vi "CSM_ExampleBrowser.vi"() -> ()   [LabVIEW 2017, in "CSM_ExampleBrowser.lvlib"]
uses:
  CSM_ExampleBrowser.lvlib
  controls/BMark_UI Data.ctl
  <vilib>/addons/analyzer/_analyzerctrls.llb/VIAnCtl Analysis App Info.ctl
  controls/BMark_Bookmark Data.ctl
  controls/BMark_VI_Identifier.ctl
  <vilib>/event_ctls.llb/eventvkey.ctl
  <vilib>/Utility/miscctls.llb/LVPoint32TypeDef.ctl
  4b753ef9-0da6-4ee4-b2e8-a0e51625f9fb.vi
  <vilib>/Array/Sort 2D Array - Pop Stack.vi
  <vilib>/Array/Sort 2D Array - Push Stack.vi
  globals/BMark_User Visible Strings.vi
  <userlib>/_OpenG.lib/string/string.llb/Convert EOLs (String)__ogtk.vi
  _Shared/CSM Shared.lvlib
  Communicable State Machine.lvlib
  _Support/csm-tool-support.lvlib
panel:
  in  "BookmarkTree":string(tree)
  in  "Refresh":bool
  in  "Zoom Factor":dbl(slide)=0.1 min=0.1 max=1.0 step=0.001 scale=0.1..1.0
  out "Warning glyph":bool
  in  "ExampleTree":string(tree)
  in  "BookmarkList":i32(listbox)
  out "String":string
  out "Preview":picture
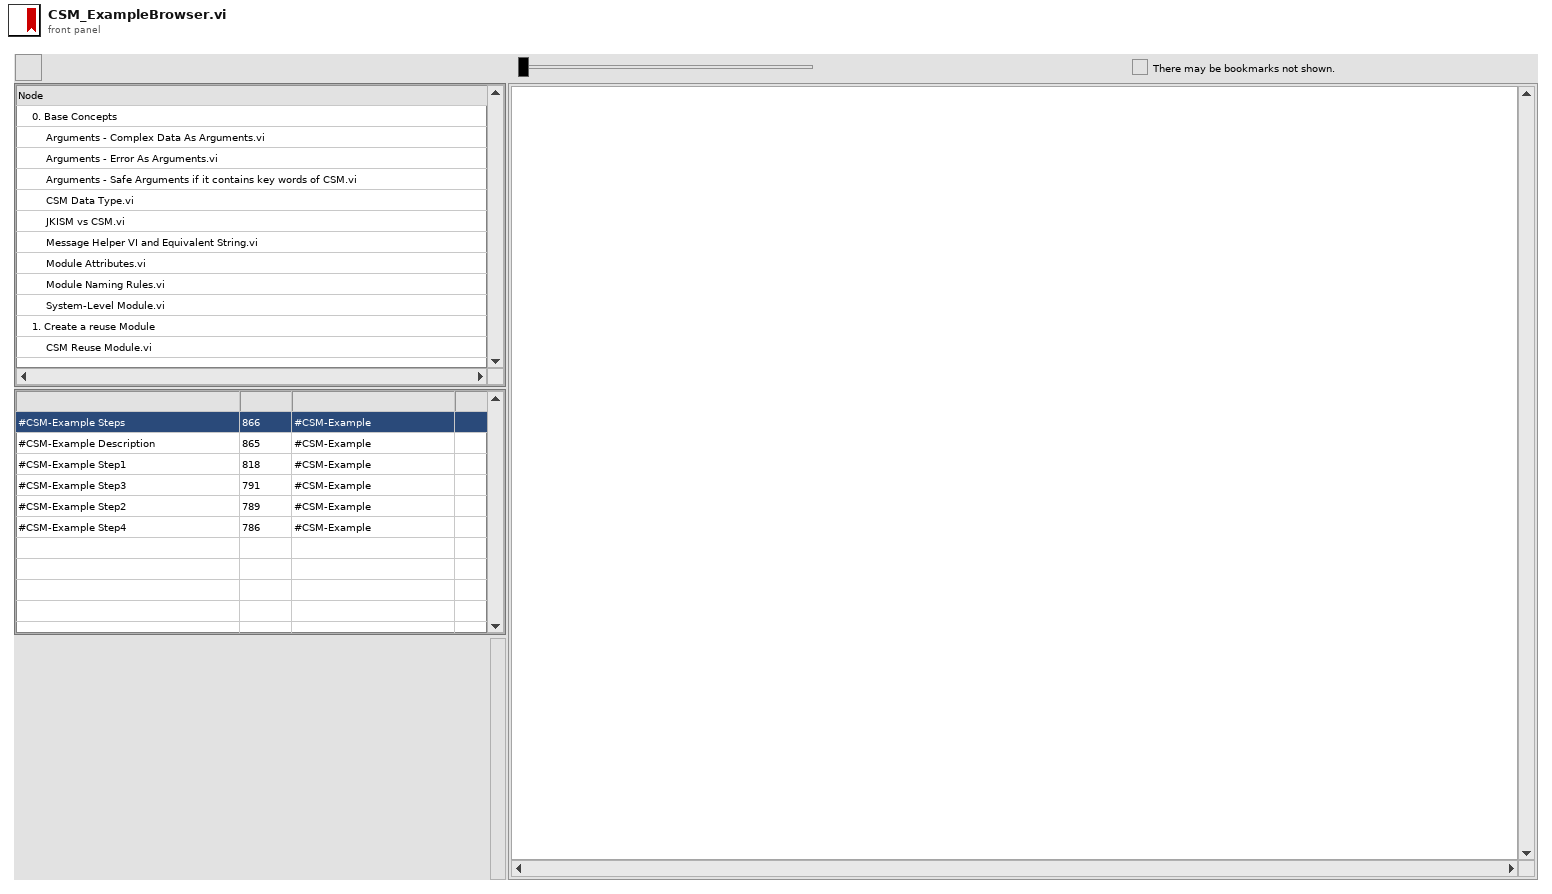
[diagram p1: front panel]
types:
  T1 = typedef "BMark_UI Data.ctl" = cluster{"Tree":refnum<vi>, "Warning glyph":refnum<vi>, "More information":refnum<vi>, "Front Panel":refnum<vi>, "GroupByVI":bool, "all projects":T2[], "bookmarks":T3[], "App Info":T2, "Preview image":refnum<vi>}
  T2 = typedef "VIAnCtl Analysis App Info.ctl" = cluster{"Project Name":string, "Target Name":string}
  T3 = typedef "BMark_Bookmark Data.ctl" = cluster{"bookmark tag":string, "full text":string, "bookmark ref":i32, "VI display name":string, "VI identifier":T4}
  T4 = typedef "BMark_VI_Identifier.ctl" = cluster{"Name":string, "Path":path, "App Info":T2}
  T5 = typedef "eventvkey.ctl" = enum16{"ASCII", "Enter", "Return", "Shift", "Ctrl", "Alt", "Cmd", "Opt", "Caps", "NumLock", "Clear", "Break", "Up", "Down", "Left", "Right", "Insert", "Delete", "Home", "End", "PageUp", "PageDown", "Escape", "Help", "Pause", "ScrollLock", "F1", "F2", "F3", "F4", "F5", "F6", "F7", "F8", "F9", "F10", "F11", "F12", "F13", "F14", "F15", "F16", "F17", "F18", "F19", "F20", "F21", "F22", "F23", "F24", "Play", "VolumeUp", "VolumeDown", "Mute", "Two Byte Char"}
  T6 = enum32{"Invalid", "Standard", "Closed", "Hidden", "Minimized", "Maximized"}
  T7 = enum32{"invalid app kind", "Development System", "Run Time System", "Student Edition", "Embedded LabVIEW", "Evaluation", "Custom"}
  T8 = enum8{"Enabled", "Disabled", "Disabled and Grayed Out"}
  T9 = typedef "LVPoint32TypeDef.ctl" = cluster{"Horizontal":i32, "Vertical":i32}
  T10 = typedef "LVPointTypeDef.ctl" = cluster{"Horizontal":i16, "Vertical":i16}
  T11 = cluster{"Core":cluster{"Current VI Reference":refnum<vi>, "Close Panel on Exit?":bool}, "root":path, "PreviewMouseDown":bool, "PreviewMouseDownCoords":T9, "PreviewMouseDownOrigin":T9}
  T12 = typedef "LVRectTypeDef.ctl" = cluster{"Left":i16, "Top":i16, "Right":i16, "Bottom":i16}
  T13 = cluster{"Current VI Reference":refnum<vi>, "Close Panel on Exit?":bool}
  T14 = typedef "LVBookmarkInfoTypeDef.ctl" = cluster{"Bookmark Reference":u32, "Bookmark Tag":string, "Label Text":string}[]
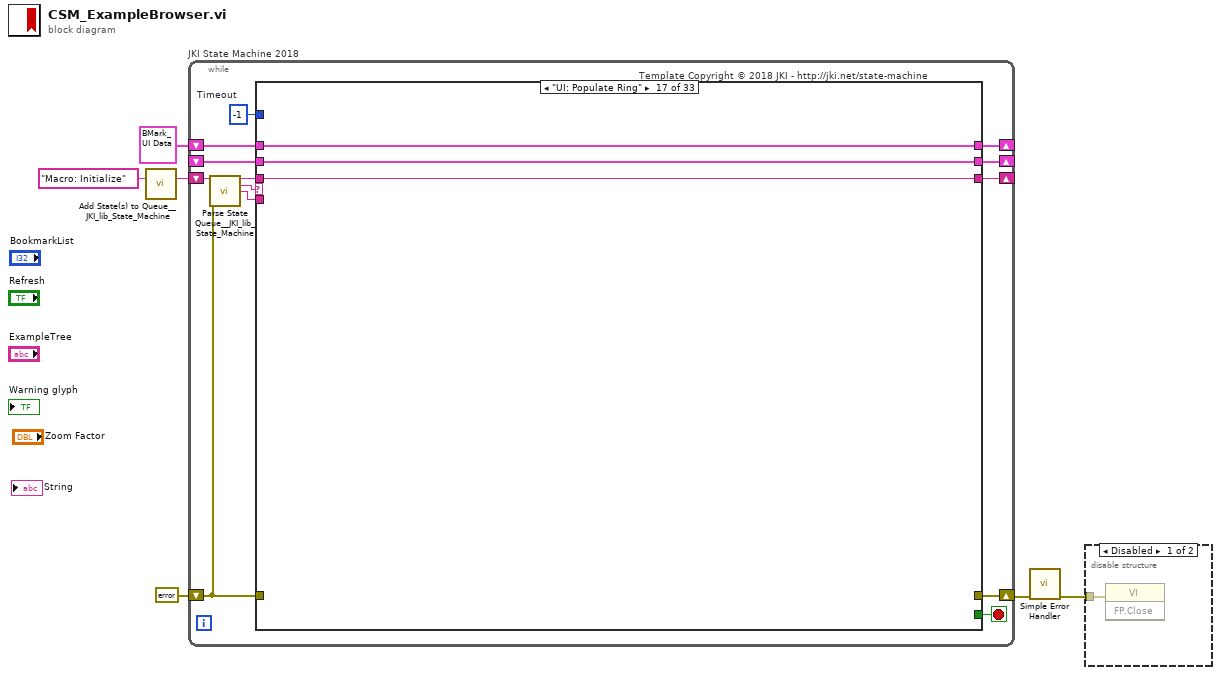
[diagram p0: block diagram]
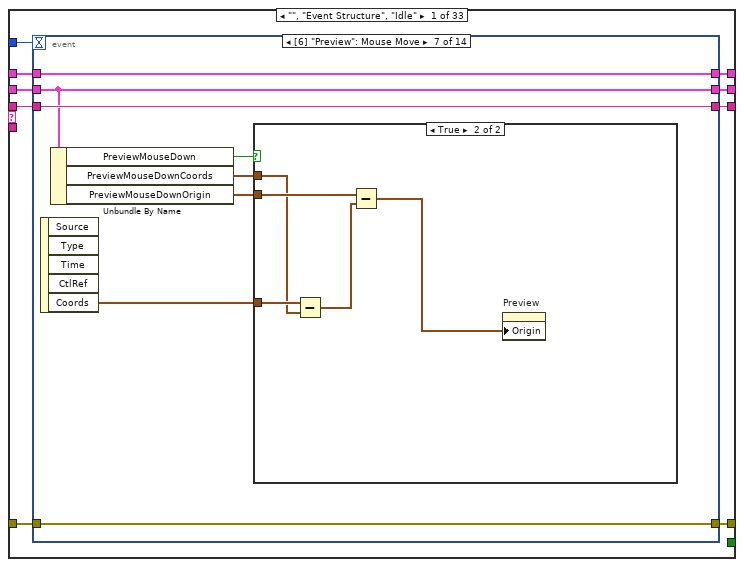
[diagram p2: hidden frame]
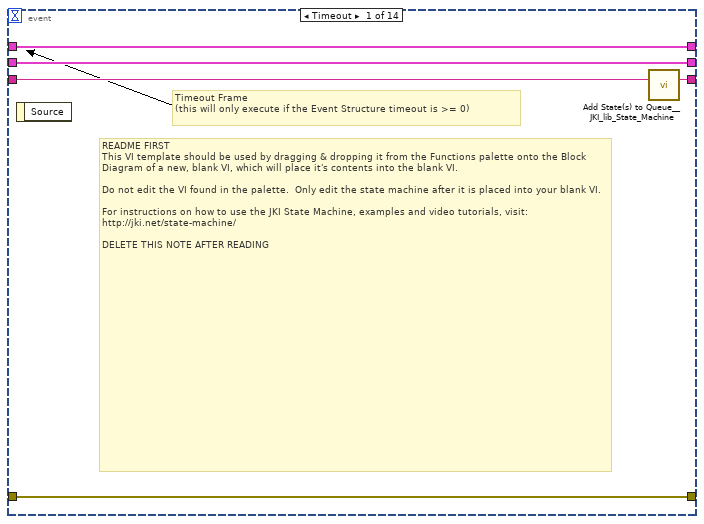
[diagram p3: hidden frame]
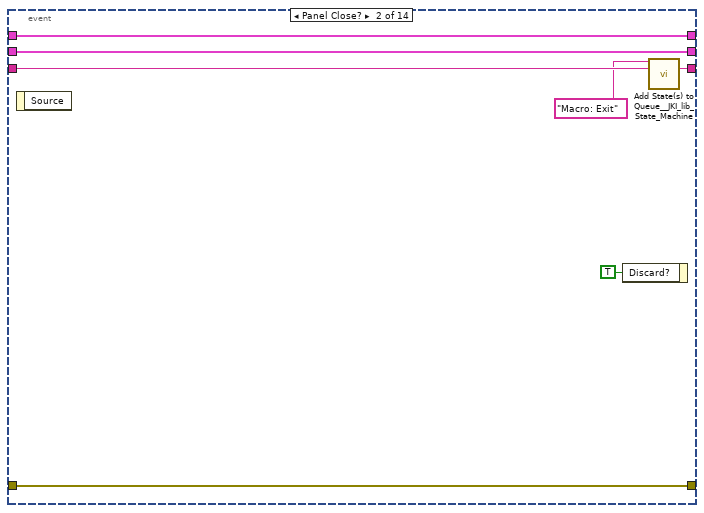
[diagram p4: hidden frame]
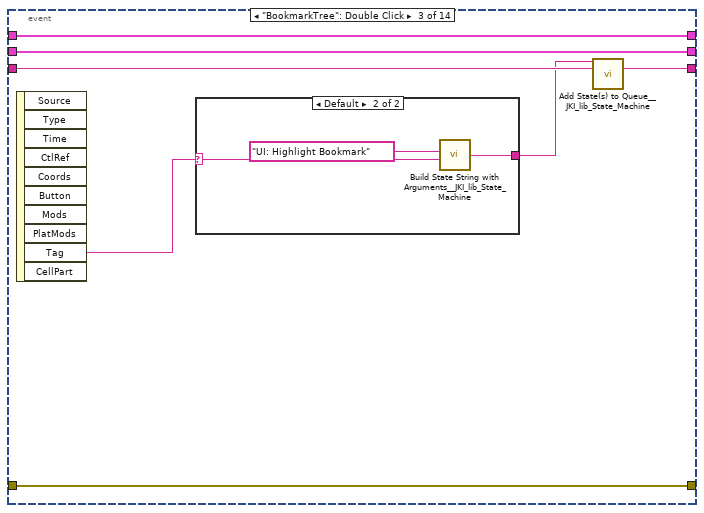
[diagram p5: hidden frame]
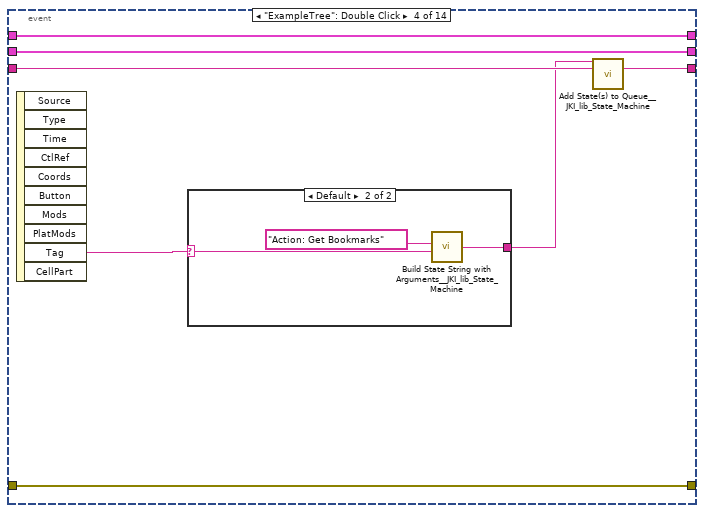
[diagram p7: hidden frame]
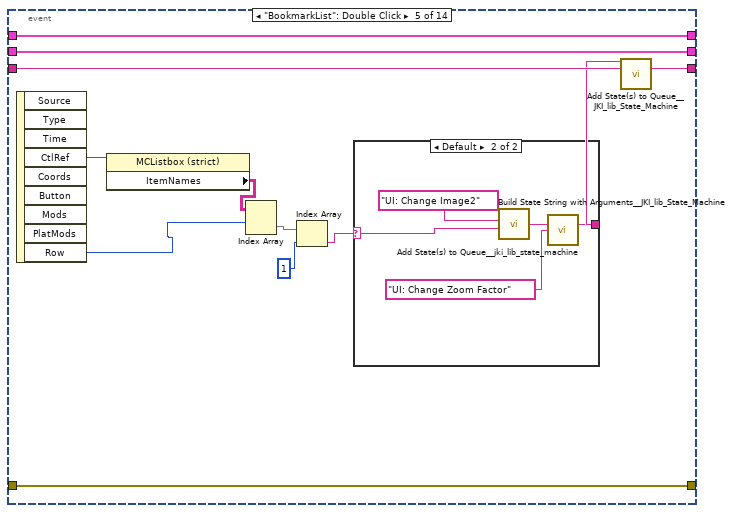
[diagram p9: hidden frame]
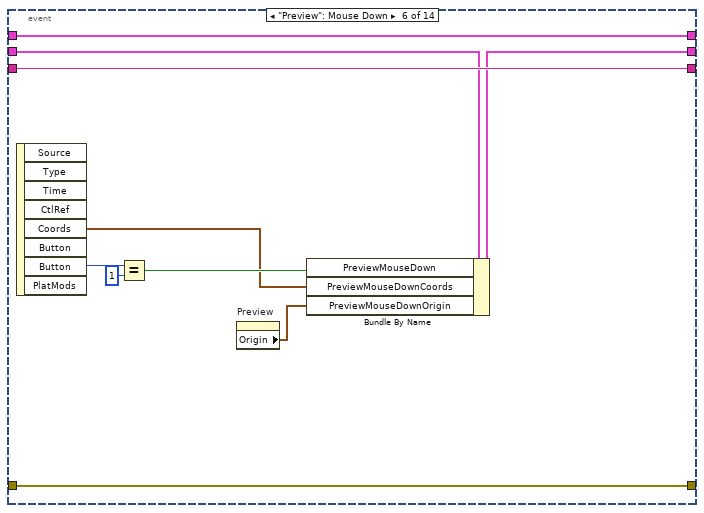
[diagram p11: hidden frame]
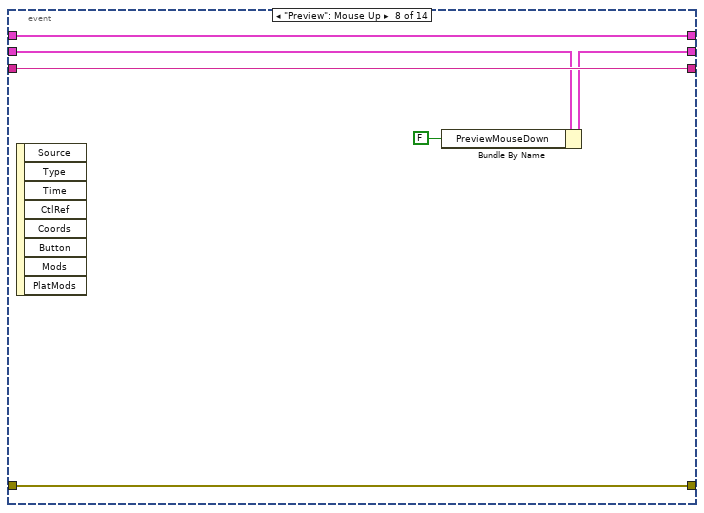
[diagram p13: hidden frame]
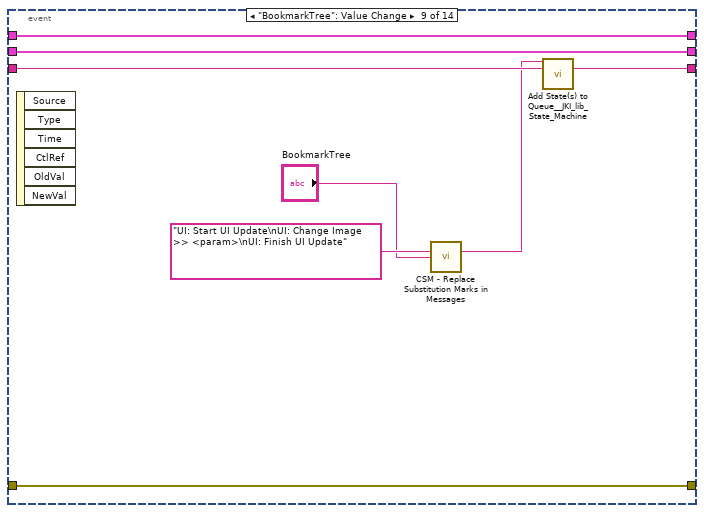
[diagram p14: hidden frame]
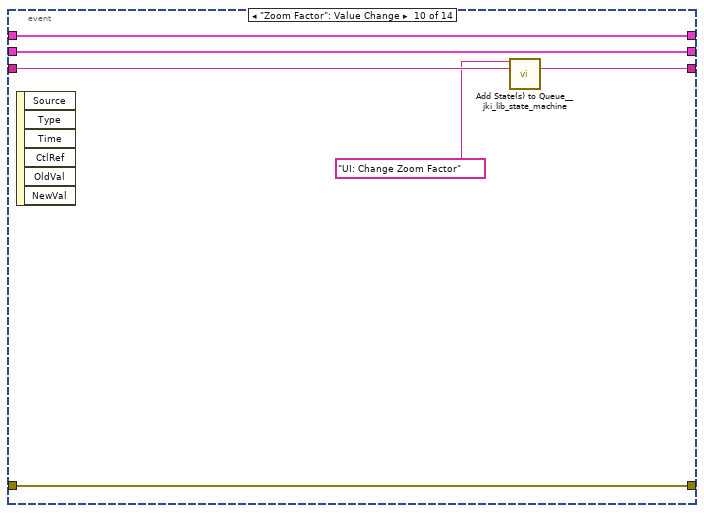
[diagram p15: hidden frame]
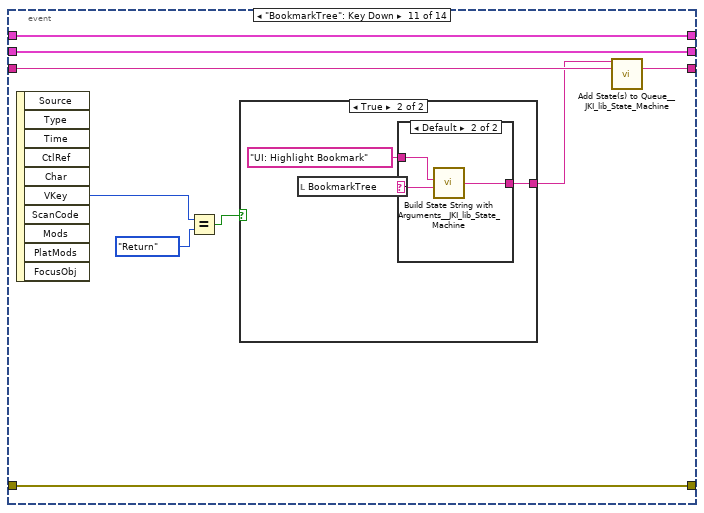
[diagram p16: hidden frame]
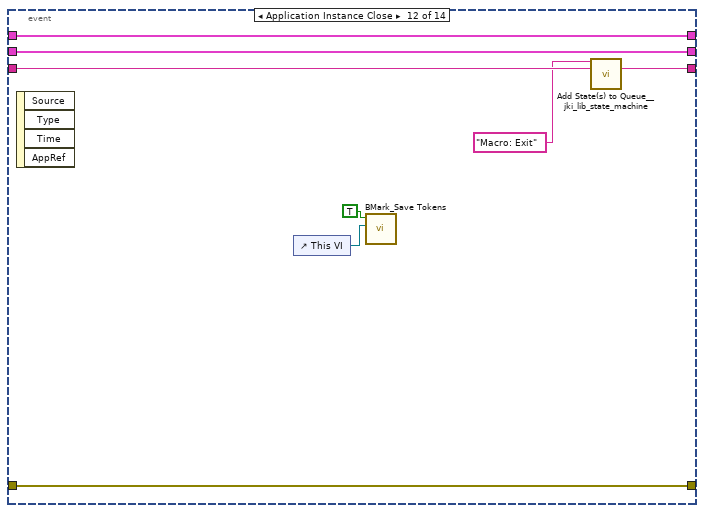
[diagram p19: hidden frame]
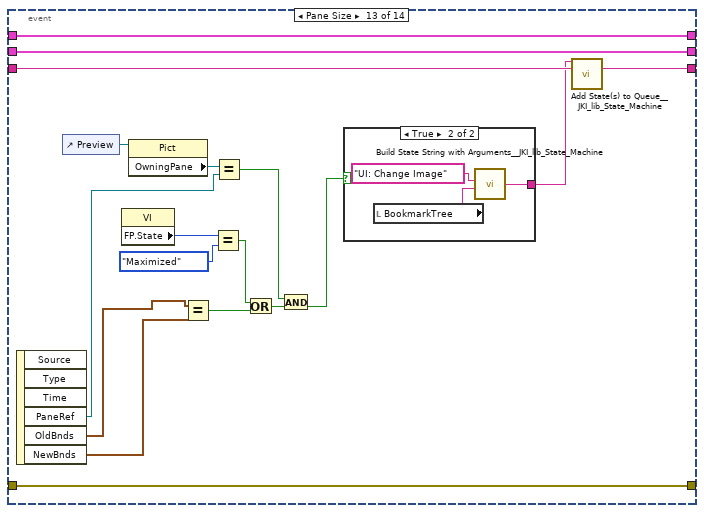
[diagram p20: hidden frame]
diagram:
  n1 = call <vilib>:"Add State(s) to Queue__JKI_lib_State_Machine.vi"("State(s) in (\"\")"="Macro: Initialize") -> ("States Out"=w4:string)  [unwired: 14 in]
  n2 = while "JKI State Machine 2018" {
    shift-right: [w12] -> _
    shift-left: _ -> [w11]
    shift-right: [w15] -> w1
    shift-left: errorcluster {"status"=FALSE, "code"=0, "source"=""} ("error out") -> [w9]
    shift-right: [w14] -> _
    shift-left: w4 -> [w16]
    shift-right: [w8] -> _
    shift-left: T1 {"Tree"=refnum, "Warning glyph"=refnum, "More information"=refnum, "Front Panel"=refnum, "GroupByVI"=FALSE, "all projects"=[], "bookmarks"=[], "App Info"={"Project Name"="", "Target Name"=""}, "Preview image"=refnum} ("Data Cluster") -> [w7]
    stop <- w13 stop-if-true
    w10 = -1  # Timeout
    # "Template Copyright © 2018 JKI - http://jki.net/state-machine"
    n3 = call <vilib>:"Parse State Queue__JKI_lib_State_Machine.vi"("State Queue"=w16, "Error In (no error)"=w9) -> ("Remaining States"=w18:string, "Current State"=w19:string, "Arguments"=w17:string)  [unwired: 11 in]
    n4 = case shown="\"UI: Populate Ring\"" w19 {
      selector: w19 -> [_ _ w177 _ _ _ _ _ _ _ _ _ _ _ _ _ _ _ _ _ _ _ _ _ _ _ _ _ _ _ _ _ _]
      tunnel: w18 -> [w28 w175 w181 w201 w208 w214 w219 w240 w247 w252 w262 w264 w284 w293 w302 w313 w316 w331 w340 w356 w370 w380 w383 w401 w413 w484 w493 w499 w510 w515 w520 w531 w548]
      tunnel: w17 -> [_ _ _ _ _ _ _ _ _ _ _ _ _ w291 _ _ _ _ _ w342 w368 w372 w385 w396 w407 w480 _ _ _ _ _ w527 _]
      tunnel: w11 -> [w26 w172 w179 w194 w205 w212 w216 _ w242 w249 w260 w273 w283 w296 w301 w312 w315 w320 w339 w355 w369 w376 w394 w399 w409 w483 w490 w496 w507 w512 w517 w529 w545]
      tunnel: [w25 w173 w183 w198 errorcluster {"status"=FALSE, "code"=0, "source"=""} ("error out") w211 w217 w237 w243 w250 w259 w267 w285 w297 w303 w304 _ w319 w341 w345 _ _ w381 w397 w410 w485 w491 w497 w508 w513 w518 w532 w546] -> w15
      tunnel: w9 -> [w24 w173 w182 w198 w204 w211 w217 w237 w244 w250 w259 _ w285 w297 w303 _ _ _ w341 _ _ _ _ w398 w411 w485 w491 w497 w508 w513 w518 w532 w546]
      tunnel: [w27 w174 w180 w200 w207 w213 w218 w239 w246 w251 w261 w265 w284 w294 w302 w313 w316 w331 w340 w356 w370 w380 w384 w400 w412 w484 w492 w498 w509 w514 w519 w531 w547] -> w14
      tunnel: [_ _ _ _ _ TRUE _ _ _ _ _ _ _ _ _ _ _ _ _ _ _ _ _ _ _ _ _ _ _ _ _ _ _] -> w13
      tunnel: [w23 w172 w179 w199 w205 w212 w216 w233 w242 w249 w260 w273 w283 w296 w301 w312 w315 w320 w339 w355 w369 w376 w394 w399 w409 w483 w490 w496 w507 w512 w517 w529 w545] -> w12
      tunnel: w10 -> [w22 _ _ _ _ _ _ _ _ _ _ _ _ _ _ _ _ _ _ _ _ _ _ _ _ _ _ _ _ _ _ _ _]
      tunnel: [w21 w171 w176 w188 w202 w209 w215 w226 w241 w248 w258 w266 w274 w287 w298 w306 w314 w322 w336 w346 w367 w379 w388 w395 w406 w482 w489 w494 w500 w511 w516 w530 w544] -> w8
      tunnel: w7 -> [w20 w171 w176 w188 w202 w209 w215 w227 w241 w248 w258 w266 w274 w295 w298 w305 w314 w322 w336 w346 w367 w379 w389 w395 w406 w482 w489 w494 w500 w511 w516 w530 w544]
      frame "", "Event Structure", "Idle" {
        n5 = event shown="[6] \"Preview\": Mouse Move" {
          selector: _ -> [_ _ _ _ _ _ _ _ _ _ _ _ _ _]
          dyn-events: _ -> [_ _ _ _ _ _ _ _ _ _ _ _ _ _]
          timeout: w22 -> [_ _ _ _ _ _ _ _ _ _ _ _ _ _]
          tunnel: w28 -> [w33 w40 w43 w53 w68 w87 w95 w106 w110 w116 w123 w137 w151 w166]
          tunnel: [w32 w39 w44 w54 w69 w87 w95 w106 w111 w117 w124 w138 w152 w167] -> w27
          tunnel: w26 -> [w30 w37 w46 w56 w71 w85 w92 w104 w113 w119 w128 w142 w160 w169]
          tunnel: [w31 w38 w47 w57 w72 w86 w94 w105 w114 w120 w129 w143 w161 w170] -> w25
          tunnel: w24 -> [w31 w38 w47 w57 w72 w86 w94 w105 w114 w120 w129 w143 w161 w170]
          tunnel: [w30 w37 w46 w56 w71 w83 w92 w102 w113 w119 w128 w142 w160 w169] -> w23
          tunnel: [w29 w34 w45 w55 w70 w84 w93 w103 w112 w118 w127 w141 w159 w168] -> w21
          tunnel: w20 -> [w29 w34 w45 w55 w70 w84 w93 w103 w112 w118 w127 w141 w159 w168]
          event Timeout {
            # "README FIRST\nThis VI template should be used by dragging & dropping it from the Functions palette onto the Block Diagram of a new, blank VI, which will place it's contents into the blank VI.\n\nDo not edit the VI found in the palette.  Only edit the state machine after it is placed into your blank VI.\n\nFor instructions on how to use the JKI State Machine, examples and video tutorials, visit:\nhttp://jki.net/state-machine/\n\nDELETE THIS NOTE AFTER READING"
            # "Timeout Frame\n(this will only execute if the Event Structure timeout is >= 0)"
            n6 = event-data() -> ()  [unwired: 1 in, 1 out]
            n7 = call <vilib>:"Add State(s) to Queue__JKI_lib_State_Machine.vi"("State(s) in (\"\")"=w33) -> ("States Out"=w32:string)  [unwired: 14 in]
          }
          event Panel Close? {
            n8 = event-data() -> ()  [unwired: 1 in, 1 out]
            n9 = event-data("Discard?"=TRUE) -> ()  [unwired: 1 in, 1 out]
            n10 = call <vilib>:"Add State(s) to Queue__JKI_lib_State_Machine.vi"("State(s) in Front (\"\")"="Macro: Exit", "State(s) in (\"\")"=w40) -> ("States Out"=w39:string)  [unwired: 13 in]
          }
          event "BookmarkTree": Double Click {
            n11 = event-data() -> ("Tag"=w41:string)  [unwired: 1 in, 9 out]
            n12 = case shown="Default" w41 {
              selector: w41 -> [_ w48]
              tunnel: [_ w49] -> w42
              frame "" {
              }
              frame Default {
                n13 = call <vilib>:"Build State String with Arguments__JKI_lib_State_Machine.vi"("Arguments (\"\")"=w48, "State"="UI: Highlight Bookmark" ("Message")) -> ("State with Arguments"=w49:string)  [unwired: 4 in]
              }
            }
            n14 = call <vilib>:"Add State(s) to Queue__JKI_lib_State_Machine.vi"("State(s) in Front (\"\")"=w42, "State(s) in (\"\")"=w43) -> ("States Out"=w44:string)  [unwired: 13 in]
          }
          event "ExampleTree": Double Click {
            n15 = event-data() -> ("Tag"=w51:string)  [unwired: 1 in, 9 out]
            n16 = case shown="Default" w51 {
              selector: w51 -> [_ w58]
              tunnel: [_ w59] -> w52
              frame "" {
              }
              frame Default {
                n17 = call <vilib>:"Build State String with Arguments__JKI_lib_State_Machine.vi"("Arguments (\"\")"=w58, "State"="Action: Get Bookmarks" ("Message")) -> ("State with Arguments"=w59:string)  [unwired: 4 in]
              }
            }
            n18 = call <vilib>:"Add State(s) to Queue__JKI_lib_State_Machine.vi"("State(s) in Front (\"\")"=w52, "State(s) in (\"\")"=w53) -> ("States Out"=w54:string)  [unwired: 13 in]
          }
          event "BookmarkList": Double Click {
            n19 = event-data() -> ("CtlRef"=w66:refnum<vi>, "Row"=w64:i32)  [unwired: 1 in, 7 out]
            n20 = property class="MCListbox (strict)"(reference=w66) -> ("ItemNames"=w65:string[][])  [unwired: 1 in, 2 out]
            n21 = Index Array(array=w65, index (row)=w64) -> (element=w63:string[])  [unwired: 1 in]
            n22 = Index Array(array=w63, index=1) -> (element=w62:string)
            n23 = case shown="Default" w62 {
              selector: w62 -> [_ w76]
              tunnel: [_ w75] -> w67
              frame "" {
              }
              frame Default {
                n24 = call <vilib>:"Build State String with Arguments__JKI_lib_State_Machine.vi"("Arguments (\"\")"=w76, "State"="UI: Change Image2" ("Message")) -> ("State with Arguments"=w74:string)  [unwired: 4 in]
                n25 = call <vilib>:"Add State(s) to Queue__jki_lib_state_machine.vi"("State(s) in (\"\")"=w74, "State(s) at Back (\"\")"="UI: Change Zoom Factor" ("Message")) -> ("States Out"=w75:string)  [unwired: 13 in]
              }
            }
            n26 = call <vilib>:"Add State(s) to Queue__JKI_lib_State_Machine.vi"("State(s) in Front (\"\")"=w67, "State(s) in (\"\")"=w68) -> ("States Out"=w69:string)  [unwired: 13 in]
          }
          event "Preview": Mouse Down {
            n27 = event-data() -> ("Coords"=w79:T9, "Button"=w82:u16)  [unwired: 1 in, 6 out]
            n28 = Equal?(x=w82, y=u16 1) -> (x = y?=w81:bool)
            n29 = property on="Preview" class="Pict"() -> ("Origin"=w78:T10)  [unwired: 2 in, 2 out]
            n30 = Bundle By Name(cluster=w85, "PreviewMouseDown"=w81, "PreviewMouseDownCoords"=w79, "PreviewMouseDownOrigin"=w78) -> (w83:T11)
          }
          event "Preview": Mouse Move {
            n31 = event-data() -> ("Coords"=w89:T9)  [unwired: 1 in, 4 out]
            n32 = Unbundle By Name(w92) -> ("PreviewMouseDown"=w91:bool, "PreviewMouseDownCoords"=w90:T9, "PreviewMouseDownOrigin"=w88:T9)
            n33 = case shown="True" w91 {
              tunnel: w90 -> [_ w98]
              tunnel: w89 -> [_ w99]
              tunnel: w88 -> [_ w100]
              frame False {
              }
              frame True {
                n34 = Subtract(x=w99, y=w98) -> (x-y=w97:T9)
                n35 = Subtract(x=w100, y=w97) -> (x-y=w96:T9)
                n36 = property on="Preview" class="Pict"("Origin"=w96) -> ()  [unwired: 2 in, 2 out]
              }
            }
          }
          event "Preview": Mouse Up {
            n37 = event-data() -> ()  [unwired: 1 in, 8 out]
            n38 = Bundle By Name(cluster=w104, "PreviewMouseDown"=FALSE) -> (w102:T11)
          }
          event "BookmarkTree": Value Change {
            n39 = event-data() -> ()  [unwired: 1 in, 6 out]
            n40 = call "CSM - Replace Substitution Marks in Messages.vi"("States With Replace Token"="UI: Start UI Update\nUI: Change Image >> <param>\nUI: Finish UI Update" ("State(s) in Front (\"\")"), "<param>"="BookmarkTree") -> ("States"=w108:string)  [unwired: 13 in]
            n41 = call <vilib>:"Add State(s) to Queue__JKI_lib_State_Machine.vi"("State(s) in Front (\"\")"=w108, "State(s) in (\"\")"=w110) -> ("States Out"=w111:string)  [unwired: 13 in]
          }
          event "Zoom Factor": Value Change {
            n42 = event-data() -> ()  [unwired: 1 in, 6 out]
            n43 = call <vilib>:"Add State(s) to Queue__jki_lib_state_machine.vi"("State(s) in Front (\"\")"="UI: Change Zoom Factor" ("State(s) in Front (\"\")"), "State(s) in (\"\")"=w116) -> ("States Out"=w117:string)  [unwired: 13 in]
          }
          event "BookmarkTree": Key Down {
            n44 = event-data() -> ("VKey"=w125:T5)  [unwired: 1 in, 9 out]
            n45 = Equal?(x=w125, y=eventvkey."Return") -> (x = y?=w122:bool)
            n46 = case shown="True" w122 {
              tunnel: [_ w130] -> w121
              frame False {
              }
              frame True {
                n47 = local read "BookmarkTree"() -> (w132:string)
                n48 = case shown="Default" w132 {
                  selector: w132 -> [_ w134]
                  tunnel: [_ w135] -> w130
                  tunnel: "UI: Highlight Bookmark" ("Message") -> [_ w133]
                  frame "" {
                  }
                  frame Default {
                    n49 = call <vilib>:"Build State String with Arguments__JKI_lib_State_Machine.vi"("Arguments (\"\")"=w134, "State"=w133) -> ("State with Arguments"=w135:string)  [unwired: 4 in]
                  }
                }
              }
            }
            n50 = call <vilib>:"Add State(s) to Queue__JKI_lib_State_Machine.vi"("State(s) in Front (\"\")"=w121, "State(s) in (\"\")"=w123) -> ("States Out"=w124:string)  [unwired: 13 in]
          }
          event Application Instance Close {
            n51 = event-data() -> ()  [unwired: 1 in, 4 out]
            n52 = control-ref of="This VI"() -> (w140:refnum<vi>)
            n53 = call "BMark_Save Tokens.vi"("reference"=w140, "GroupByVI"=TRUE) -> ()  [unwired: 10 in]
            n54 = call <vilib>:"Add State(s) to Queue__jki_lib_state_machine.vi"("State(s) in Front (\"\")"="Macro: Exit" ("State(s) in Front (\"\")"), "State(s) in (\"\")"=w137) -> ("States Out"=w138:string)  [unwired: 13 in]
          }
          event Pane Size {
            n55 = event-data() -> ("PaneRef"=w146:refnum<vi>, "OldBnds"=w154:T12, "NewBnds"=w153:T12)  [unwired: 1 in, 3 out]
            n56 = control-ref of="Preview"() -> (w148:refnum<vi>)
            n57 = property class="VI"() -> ("FP.State"=w158:T6)  [unwired: 2 in, 2 out]
            n58 = property class="Pict"(reference=w148) -> ("OwningPane"=w147:refnum<vi>)  [unwired: 1 in, 2 out]
            n59 = Equal?(x=w154, y=w153) -> (x = y?=w155:bool)
            n60 = Equal?(x=w158, y=T6."Maximized" ("Front Panel Window:State")) -> (x = y?=w156:bool)
            n61 = Equal?(x=w147, y=w146) -> (x = y?=w144:bool)
            n62 = Or(x=w156, y=w155) -> (x .or. y?=w149:bool)
            n63 = And(x=w144, y=w149) -> (x .and. y?=w145:bool)
            n64 = case shown="True" w145 {
              tunnel: [_ w162] -> w150
              frame False {
              }
              frame True {
                n65 = local read "BookmarkTree"() -> (w163:string)
                n66 = call <vilib>:"Build State String with Arguments__JKI_lib_State_Machine.vi"("Arguments (\"\")"=w163, "State"="UI: Change Image" ("Message")) -> ("State with Arguments"=w162:string)  [unwired: 4 in]
              }
            }
            n67 = call <vilib>:"Add State(s) to Queue__JKI_lib_State_Machine.vi"("State(s) in Front (\"\")"=w150, "State(s) in (\"\")"=w151) -> ("States Out"=w152:string)  [unwired: 13 in]
          }
          event event #0x52 {
            n68 = event-data() -> ()  [unwired: 1 in, 6 out]
            n69 = call <vilib>:"Add State(s) to Queue__jki_lib_state_machine.vi"("State(s) in Front (\"\")"="UI: Clear Tree\nUI: Start UI Update\nUI: Populate Ring\nUI: Populate Tree\nUI: Finish UI Update " ("State(s) in Front (\"\")"), "State(s) in (\"\")"=w166) -> ("States Out"=w167:string)  [unwired: 13 in]
          }
        }
      }
      frame "---------- Core ----------" {
        # "Do not put any code in this frame.\n(it is a separator no-op)"
        n70 = call <vilib>:"Add State(s) to Queue__JKI_lib_State_Machine.vi"("State(s) in (\"\")"=w175) -> ("States Out"=w174:string)  [unwired: 14 in]
      }
      frame Default {
        w186 = 42 items=["No error", "Argument error", "Memory is full", "Out of zone", "End of file", "File already open", "Generic file I/O error", "File not found", "File permission error", "Disk is full", "Duplicate path", "Too many files open", "System feature not enabled", "Resource file not found", "Cannot add resource", "Resource not found", "Image not found", "Image memory error", "Pen does not exist", "Config type invalid", "Config token not found", "Config parse error", "Config memory error", "Bad external code format", "Bad external code offset", "External code not present", "Null window", "Destroy window error", "Null menu", "Print aborted", "Bad print record", "Print driver error", "Windows error during printing", "Memory error during printing", "Print dialog error", "Generic print error", "Invalid device refnum", "Device not found", "Device parameter error", "Device unit error", "Cannot open device", "Device call aborted", "Generic error", "Cancelled by user", "Object ID too low", "Object ID too high", "Object not in heap", "Unknown heap", "Unknown object (invalid DefProc)", "Unknown object (DefProc not in table)", "Message out of range", "Invalid (null) method", "Unknown message", "Manager call not supported", "Bad address", "Network operation in progress", "Network operation timed out", "Connection is busy", "Network attribute not supported", "Network error", "Address in use", "System out of memory", "Connection aborted", "Connection refused", "Not connected", "Already connected", "Connection closed", "Initialization error (interapplication manager)", "Bad occurrence", "Wait on unbound occurrence handler", "Occurrence queue overflow", "Datalog type conflict", "Unused", "Unrecognized type (interapplication manager)", "Memory corrupt", "Failed to make temporary DLL", "Old CIN version", "Drag socket not found", "Failed to load drop-object", "Failed to register OLE object", "Failed to release OLE object", "Format specifier type mismatch", "Unknown format specifier", "Too few format specifiers", "Too many format specifiers", "Scan failed", "Newer CIN version", "Error converting to variant", "Runtime menu error", "Password tampered", "Variant attribute not found", "Incompatible variant data type", "Event data is not available", "Event Store is not present", "Occurrence is not found", "Event Queue is not created", "Event info is not available", "Refnum passed is NULL", "Error retrieving Class GUID", "Error retrieving CoClass GUID", "Error retrieving TypeLib GUID.", "Bad built application magic bytes.", "Specific driver is different from the specific driver associated with the Logical Name.", "There is no session opened to the class driver.", "Max Error", "MAX - Error with config objects", "MAX - Error loading configuration", "MAX - Group not supported"]
        # "Current State"
        # "Do not delete, rename, or modify this frame.\n(this is used to capture unhandled states and typos)"
        # "Handle mistyped state name (developer tool)"
        n71 = Format Into String(format string="Software Exception: Unhandled State \"%s\"." ("message"), error in=w182, w177) -> (resulting string=w185:string, error out=w184:errorcluster)  [unwired: 1 in]
        n72 = call <vilib>:"Error Cluster From Error Code.vi"("show call chain? (False)"=TRUE, "error in (no error)"=w184, "error message (\"\")"=w185, "error code (0)"=w186) -> ("error out"=w183:errorcluster)  [unwired: 5 in]
        n73 = call <vilib>:"Add State(s) to Queue__JKI_lib_State_Machine.vi"("State(s) in (\"\")"=w181) -> ("States Out"=w180:string)  [unwired: 14 in]
      }
      frame "Initialize Core Data" {
        # "Do not delete, rename, or modify this frame.\n(this is used to determine panel behavior on exit)"
        # "originally closed?"
        # "exe?"
        # "If panel starts closed or is an EXE, then close it when we exit"
        n74 = property class="VI"() -> ("FP.State"=w191:T6)  [unwired: 2 in, 2 out]
        n75 = property class="App"() -> ("App.Kind"=w197:T7)  [unwired: 2 in, 2 out]
        n76 = control-ref of="Current VI Reference"() -> (w192:refnum<vi>)
        n77 = Equal?(x=w191, y=T6."Closed" ("Front Panel Window:State")) -> (x = y?=w189:bool)
        n78 = Equal?(x=w197, y=T7."Run Time System" ("Application:Kind")) -> (x = y?=w195:bool)
        n79 = Or(x=w189, y=w195) -> (x .or. y?=w193:bool)
        n80 = Bundle By Name(cluster=w194, "Core.Current VI Reference"=w192, "Core.Close Panel on Exit?"=w193) -> (w199:T11)
        n81 = call <vilib>:"Add State(s) to Queue__JKI_lib_State_Machine.vi"("State(s) in (\"\")"=w201) -> ("States Out"=w200:string)  [unwired: 14 in]
      }
      frame "Error Handler" {
        # "Unhandled Error -- Display it"
        # "Handle any errors here.\nYou can also output any states to clean-up after errors occur"
        # "Clear error"
        n82 = call <vilib>:"General Error Handler.vi"("error in (no error)"=w204) -> ()  [unwired: 10 in, 5 out]
        n83 = call <vilib>:"Add State(s) to Queue__JKI_lib_State_Machine.vi"("State(s) in Front (\"\")"="/* Post Error States", "State(s) in (\"\")"=w208) -> ("States Out"=w207:string)  [unwired: 13 in]
      }
      frame "Exit" {
        # "Do not put any code in this frame.\n(No errors that occur here will be handled.)"
        n84 = call <vilib>:"Add State(s) to Queue__JKI_lib_State_Machine.vi"("State(s) in (\"\")"=w214) -> ("States Out"=w213:string)  [unwired: 14 in]
      }
      frame "---------- Data ----------" {
        # "Do not put any code in this frame.\n(It is a separator no-op. You can make a copy of this frame to create a new Data frame)"
        n85 = call <vilib>:"Add State(s) to Queue__JKI_lib_State_Machine.vi"("State(s) in (\"\")"=w219) -> ("States Out"=w218:string)  [unwired: 14 in]
      }
      frame "Data: Initialize" {
        w220 = T9 {"Horizontal"=0, "Vertical"=0}  # PreviewMouseDownOrigin
        w221 = T9 {"Horizontal"=0, "Vertical"=0}  # PreviewMouseDownCoords
        w222 = FALSE  # PreviewMouseDown
        w236 = T13 {"Current VI Reference"=refnum, "Close Panel on Exit?"=FALSE}  # Core
        w231 = path ""  # root
        # "Initialize the shift-register data, here.\n(data names are defined by what you wire into the bundle function)"
        n86 = property class="VI"() -> ("Panel"=w229:refnum<vi>)  [unwired: 2 in, 2 out]
        n87 = control-ref of="BookmarkTree"() -> (w228:refnum<vi>)
        n88 = control-ref of="Preview"() -> (w230:refnum<vi>)
        n89 = control-ref of="Warning glyph"() -> (w223:refnum<vi>)
        n90 = call <resource>:"LV Config Read Boolean.vi"("key"="BookmarkManager.GroupByVI") -> ("value"=w224:bool)  [unwired: 4 in, 2 out]
        n91 = Bundle By Name(cluster=w227, "Tree"=w228, "Warning glyph"=w223, "Front Panel"=w229, "Preview image"=w230, "GroupByVI"=w224) -> (w226:T1)
        n92 = Bundle("Core"=w236, "root"=w231, "PreviewMouseDown"=w222, "PreviewMouseDownCoords"=w221, "PreviewMouseDownOrigin"=w220) -> (w238:T11)  [unwired: 1 in]
        n93 = call "CSM - user.lib Dir.vi"() -> ("<LabVIEW>"=w235:path)  [unwired: 2 in, 1 out]
        n94 = Build Path(base path=w235, name or relative path="Example") -> (appended path=w232:path)
        n95 = Bundle By Name(cluster=w238, "root"=w232) -> (w233:T11)
        n96 = call <vilib>:"Add State(s) to Queue__JKI_lib_State_Machine.vi"("State(s) in (\"\")"=w240) -> ("States Out"=w239:string)  [unwired: 14 in]
      }
      frame "Data: Cleanup" {
        # "Cleanup any data and references, here.\n(this is called automatically, by the Macro: Exit)"
        n97 = Unbundle By Name(w242) -> ("Core.Current VI Reference"=w245:refnum<vi>)
        n98 = Close Reference(reference=w245, error in (no error)=w244) -> (error out=w243:errorcluster)
        n99 = call <vilib>:"Add State(s) to Queue__JKI_lib_State_Machine.vi"("State(s) in (\"\")"=w247) -> ("States Out"=w246:string)  [unwired: 14 in]
      }
      frame "---------- UI ----------" {
        # "Do not put any code in this frame.\n(It is a separator no-op. You can make a copy of this frame to create a new UI frame)"
        n100 = call <vilib>:"Add State(s) to Queue__JKI_lib_State_Machine.vi"("State(s) in (\"\")"=w252) -> ("States Out"=w251:string)  [unwired: 14 in]
      }
      frame "UI: Initialize" {
        n101 = control-ref of="Refresh"() -> (w257:refnum<vi>)
        n102 = control-ref of="Zoom Factor"() -> (w254:refnum<vi>)
        n103 = control-ref of="Splitter"() -> (w255:refnum<vi>)
        n104 = Build Array(w257, w254) -> (w256:refnum<vi>[])
        n105 = local write "Zoom Factor"(0.8 ("Zoom Factor")) -> ()
        n106 = call "Relocate Splitter Posistion.vi"("Array"=w256, "Splitter in"=w255) -> ()  [unwired: 9 in, 1 out]
        n107 = call <vilib>:"Add State(s) to Queue__JKI_lib_State_Machine.vi"("State(s) in (\"\")"=w262) -> ("States Out"=w261:string)  [unwired: 14 in]
      }
      frame "UI: Initialize Panel" {
        n108 = Unbundle By Name(w266) -> ("Tree"=w271:refnum<vi>)
        n109 = property class="Tree (strict)"(reference=w271, "ActiveColNum"=1 ("Active Cell:Active Column Number"), "Width"=4000 ("Active Cell:Cell Size:Width")) -> ()  [unwired: 1 in, 2 out]
        n110 = control-ref of="This VI"() -> (w269:refnum<vi>)
        n111 = call "BMark_OpenWindow.vi"("Bookmark manager window reference"=w269) -> ("error out"=w268:errorcluster)  [unwired: 8 in, 2 out]
        n112 = call <vilib>:"Set Busy.vi"("error in (no error)"=w268) -> ("error out"=w267:errorcluster)  [unwired: 9 in, 1 out]
        n113 = call <vilib>:"Add State(s) to Queue__JKI_lib_State_Machine.vi"("State(s) in (\"\")"=w264, "State(s) at Back (\"\")"="UI: Clear Tree\nUI: Populate Ring\nUI: Group By Changed " ("State(s) at Back (\"\")")) -> ("States Out"=w265:string)  [unwired: 13 in]
      }
      frame "UI: Clear Tree" {
        n114 = Unbundle By Name(w274) -> ("Tree"=w277:refnum<vi>)
        n115 = invoke class="Tree (strict)" method="Edit Tree Items.Delete"(reference=w277, "Delete Children"=TRUE ("Delete Children?")) -> (reference out=w278:refnum<vi>, error out=w279:errorcluster)  [unwired: 3 in, 3 out]
        n116 = global read "BMark_User Visible Strings.vi" "Populating list"() -> (w280:string)
        n117 = invoke class="Tree (strict)" method="Edit Tree Items.Add Item"(reference=w278, error in=w279, "Left Cell"=w280) -> (reference out=w281:refnum<vi>, error out=w282:errorcluster)  [unwired: 6 in, 7 out]
        n118 = property class="Tree (strict)"(reference=w281, error in=w282, "DisabledEnum"=T8."Disabled" ("Disabled")) -> ()  [unwired: 2 out]
      }
      frame "UI: Group By Changed" {
        n119 = call "CSM - Convert HexStr to Data.vi"("HEX String"=w291) -> ("Variant"=w289:variant, "error out"=w288:errorcluster)  [unwired: 7 in]
        n120 = Variant To Data(error in=w288, type=FALSE, Variant=w289) -> (data=w286:bool)  [unwired: 1 out]
        n121 = Bundle By Name(cluster=w295, "GroupByVI"=w286) -> (w287:T1)
        n122 = call <vilib>:"Add State(s) to Queue__JKI_lib_State_Machine.vi"("State(s) in (\"\")"=w293, "State(s) at Back (\"\")"="UI: Clear Tree\nUI: Start UI Update\nUI: Populate Tree\nUI: Finish UI Update" ("Message")) -> ("States Out"=w294:string)  [unwired: 13 in]
      }
      frame "UI: Start UI Update" {
        n123 = Unbundle By Name(w298) -> ("Front Panel"=w300:refnum<vi>)
        n124 = property class="Pnl"(reference=w300, "DeferPanUpdts"=TRUE ("Defer Panel Updates")) -> ()  [unwired: 1 in, 2 out]
        n125 = call <vilib>:"Set Busy.vi"() -> ()  [unwired: 10 in, 2 out]
      }
      frame "UI: Populate Tree" {
        n126 = Unbundle By Name(w305) -> ("App Info"=w310:T2, "Tree"=w309:refnum<vi>, "GroupByVI"=w308:bool)
        n127 = call "BMark_Get Bookmarks.vi"("App Info"=w310) -> ("error out"=w311:errorcluster, "bookmarks"=w307:T3[])  [unwired: 8 in, 1 out]
        n128 = call "BMark_Create Tree.vi"("error in (no error)"=w311, "GroupByVI"=w308, "TreeRef"=w309, "Bookmark info"=w307) -> ("error out"=w304:errorcluster)  [unwired: 7 in]
        n129 = Bundle By Name(cluster=w305, "bookmarks"=w307) -> (w306:T1)
      }
      frame "UI: Populate Ring" {
      }
      frame "UI: Populate Example Tree" {
        n130 = Unbundle By Name(w320) -> ("root"=w321:path)
        n131 = call <vilib>:"Recursive File List.vi"("pattern"="*.vi", "Folder Path"=w321) -> ("All Files in Dir"=w326:path[], "dup Folder Path"=w327:path)  [unwired: 5 in, 3 out]
        n132 = for {
          tunnel: w326 -> [w334] mode=indexing
          tunnel: [w332] -> w328 mode=indexing
          tunnel: w327 -> [w333]
          n133 = call <vilib>:"Compare Two Paths.vi"("Path 2"=w334, "Path 1"=w333) -> ("Relative Path from 1 to 2"=w335:path)  [unwired: 6 in, 3 out]
          n134 = Path To String(path=w335) -> (string=w332:string)
        }
        n135 = Build Array(w328) -> (w329:string[][])
        n136 = control-ref of="ExampleTree"() -> (w318:refnum<vi>)
        n137 = Transpose 2D Array(2D array=w329) -> (transposed array=w330:string[][])
        n138 = call "Populate Tree with Delimited Strings_csm.vi"("Use Child Only?"=TRUE, "Default Symbol"=26, "Delimiter"="\\", "Items (Delimited)"=w330, "Tree Control"=w318) -> ("error out"=w319:errorcluster)  [unwired: 4 in, 2 out]
      }
      frame "UI: Finish UI Update" {
        n139 = Unbundle By Name(w336) -> ("Front Panel"=w338:refnum<vi>)
        n140 = property class="Pnl"(reference=w338, "DeferPanUpdts"=FALSE ("Defer Panel Updates")) -> ()  [unwired: 1 in, 2 out]
        n141 = call <vilib>:"Unset Busy.vi"() -> ()  [unwired: 11 in, 1 out]
      }
      frame "UI: Highlight Bookmark" {
        n142 = call "CSM - Convert HexStr to Data.vi"("HEX String"=w342) -> ("Variant"=w343:variant, "error out"=w344:errorcluster)  [unwired: 7 in]
        n143 = Unbundle By Name(w346) -> ("bookmarks"=w352:T3[], "Tree"=w349:refnum<vi>)
        n144 = Variant To Data(error in=w344, type="", Variant=w343) -> (data=w351:string, error out=w353:errorcluster)
        n145 = property class="Tree (strict)"(reference=w349, error in=w353, "Active Item Tag"=w351) -> (error out=w354:errorcluster, "Indent Level"=w348:i32)  [unwired: 1 out]
        n146 = Greater Than 0?(x=w348) -> (x > 0?=w350:bool)
        n147 = case shown="True" w350 {
          tunnel: w354 -> [w357 w363]
          tunnel: [w357 w360] -> w345
          tunnel: w351 -> [_ w362]
          tunnel: w352 -> [_ w361]
          frame False {
          }
          frame True {
            n148 = call "BMark_Highlight Bookmark.vi"("error in (no error)"=w363, "bookmarks"=w361, "tag"=w362) -> ("error out"=w359:errorcluster)  [unwired: 8 in]
            n149 = call <vilib>:"Simple Error Handler.vi"("error in (no error)"=w359) -> ("error out"=w358:errorcluster)  [unwired: 4 in, 4 out]
            n150 = call <vilib>:"Clear Errors.vi"("error in (no error)"=w358) -> ("error out"=w360:errorcluster)  [unwired: 5 in, 1 out]
          }
        }
      }
      frame "UI: Change Image" {
        n151 = Unbundle By Name(w367) -> ()  [unwired: 1 out]
        n152 = call "CSM - Convert HexStr to Data.vi"("HEX String"=w368) -> ("Variant"=w365:variant, "error out"=w364:errorcluster)  [unwired: 7 in]
        n153 = Variant To Data(error in=w364, type="", Variant=w365) -> ()  [unwired: 2 out]
      }
      frame "UI: Change Image2" {
        n154 = local read "ExampleTree"() -> (w373:string)
        n155 = Unbundle By Name(w379) -> ("Preview image"=w378:refnum<vi>)
        n156 = Unbundle By Name(w376) -> ("root"=w375:path)
        n157 = Decimal String To Number(string=w372) -> (number=w371:i32)  [unwired: 2 in, 1 out]
        n158 = Build Path(base path=w375, name or relative path=w373) -> (appended path=w374:path)
        n159 = call "CSMExampleBrowser_Change Bookmark Image.vi"("Picture Control Reference"=w378, "Bookmark ID"=w371, "vi path"=w374) -> ("error out"=w377:errorcluster)  [unwired: 8 in]
        n160 = call <vilib>:"Clear Errors.vi"("error in (no error)"=w377) -> ()  [unwired: 5 in, 2 out]
      }
      frame "UI: Select Project" {
        n161 = call "CSM - Convert HexStr to Data.vi"("HEX String"=w385) -> ("Variant"=w386:variant, "error out"=w387:errorcluster)  [unwired: 7 in]
        n162 = Unbundle By Name(w389) -> ("all projects"=w392:T2[])
        n163 = Variant To Data(error in=w387, type=u16 0 ("Projects"), Variant=w386) -> (data=w391:u16, error out=w381:errorcluster)
        n164 = call "BMark_Get App From Ring Selection.vi"("all projects"=w392, "Projects"=w391) -> ("App Info"=w390:T2)  [unwired: 9 in]
        n165 = Bundle By Name(cluster=w389, "App Info"=w390) -> (w388:T1)
        n166 = call <vilib>:"Add State(s) to Queue__JKI_lib_State_Machine.vi"("State(s) in Front (\"\")"="UI: Clear Tree\nUI: Start UI Update\nUI: Populate Tree\nUI: Finish UI Update" ("State(s) in Front (\"\")"), "State(s) in (\"\")"=w383) -> ("States Out"=w384:string)  [unwired: 13 in]
      }
      frame "UI: Cursor Set" {
        # "Argument"
        # "Set and Unset Cursor Busy.\n(Usage: \"UI: Cursor Set >> Busy|Idle\")"
        n167 = case shown="\"Idle\", Default" w396 {
          tunnel: w398 -> [w403 w405]
          tunnel: [w402 w404] -> w397
          frame "Idle", Default {
            n168 = call <vilib>:"Unset Busy.vi"("error in (no error)"=w403) -> ("error out"=w402:errorcluster)  [unwired: 10 in]
          }
          frame "Busy" {
            n169 = call <vilib>:"Set Busy.vi"("error in (no error)"=w405) -> ("error out"=w404:errorcluster)  [unwired: 9 in, 1 out]
          }
        }
        n170 = call <vilib>:"Add State(s) to Queue__JKI_lib_State_Machine.vi"("State(s) in (\"\")"=w401) -> ("States Out"=w400:string)  [unwired: 14 in]
      }
      frame "UI: Front Panel State" {
        # "Argument"
        # "Set Front Panel Open or Closed\n(Usage: \"UI: Front Panel State >> Open|Close\")"
        n171 = Unbundle By Name(w409) -> ("Core.Current VI Reference"=w408:refnum<vi>)
        n172 = case shown="\"Open\", \"Standard\", Default" w407 {
          tunnel: w411 -> [w419 w434 w445 w458 w471]
          tunnel: [w421 w435 w447 w460 w473] -> w410
          tunnel: w408 -> [w420 w432 w446 w459 w472]
          frame "Open", "Standard", Default {
            w414 = T6."Standard" ("State")
            n173 = property class="VI"(reference=w420, error in=w419) -> (reference out=w417:refnum<vi>, error out=w418:errorcluster, "FP.State"=w416:T6)
            n174 = Not Equal?(x=w416, y=w414) -> (x != y?=w415:bool)
            n175 = case shown="False" w415 {
              tunnel: [w425 w427] -> w421
              tunnel: w418 -> [w424 w427]
              tunnel: w417 -> [w423 _]
              tunnel: w414 -> [w422 _]
              frame True {
                n176 = invoke class="VI" method="FP.Open"(reference=w423, error in=w424, "Activate"=TRUE, "State"=w422) -> (error out=w425:errorcluster)  [unwired: 1 in, 4 out]
              }
              frame False {
              }
            }
          }
          frame "Close", "Closed" {
            n177 = property class="VI"(reference=w432, error in=w434) -> (reference out=w431:refnum<vi>, error out=w433:errorcluster, "FP.State"=w429:T6)
            n178 = Not Equal?(x=w429, y=T6."Closed" ("Front Panel Window:State")) -> (x != y?=w428:bool)
            n179 = case shown="True" w428 {
              tunnel: [w436 w439] -> w435
              tunnel: w433 -> [w436 w438]
              tunnel: w431 -> [_ w437]
              frame False {
              }
              frame True {
                n180 = invoke class="VI" method="FP.Close"(reference=w437, error in=w438) -> (error out=w439:errorcluster)  [unwired: 1 in, 2 out]
              }
            }
          }
          frame "Hidden", "Hide" {
            w440 = T6."Hidden" ("State")
            n181 = property class="VI"(reference=w446, error in=w445) -> (reference out=w443:refnum<vi>, error out=w444:errorcluster, "FP.State"=w442:T6)
            n182 = Not Equal?(x=w442, y=w440) -> (x != y?=w441:bool)
            n183 = case shown="True" w441 {
              tunnel: [w451 w452] -> w447
              tunnel: w444 -> [w450 w452]
              tunnel: w443 -> [w449 _]
              tunnel: w440 -> [w448 _]
              frame True {
                n184 = invoke class="VI" method="FP.Open"(reference=w449, error in=w450, "State"=w448) -> (error out=w451:errorcluster)  [unwired: 2 in, 4 out]
              }
              frame False {
              }
            }
          }
          frame "Minimize", "Minimized" {
            w453 = T6."Minimized" ("State")
            n185 = property class="VI"(reference=w459, error in=w458) -> (reference out=w456:refnum<vi>, error out=w457:errorcluster, "FP.State"=w455:T6)
            n186 = Not Equal?(x=w455, y=w453) -> (x != y?=w454:bool)
            n187 = case shown="True" w454 {
              tunnel: [w464 w465] -> w460
              tunnel: w457 -> [w463 w465]
              tunnel: w456 -> [w462 _]
              tunnel: w453 -> [w461 _]
              frame True {
                n188 = invoke class="VI" method="FP.Open"(reference=w462, error in=w463, "State"=w461) -> (error out=w464:errorcluster)  [unwired: 2 in, 4 out]
              }
              frame False {
              }
            }
          }
          frame "Maximize", "Maximized" {
            w466 = T6."Maximized" ("State")
            n189 = property class="VI"(reference=w472, error in=w471) -> (reference out=w469:refnum<vi>, error out=w470:errorcluster, "FP.State"=w468:T6)
            n190 = Not Equal?(x=w468, y=w466) -> (x != y?=w467:bool)
            n191 = case shown="True" w467 {
              tunnel: [w477 w478] -> w473
              tunnel: w470 -> [w476 w478]
              tunnel: w469 -> [w475 _]
              tunnel: w466 -> [w474 _]
              frame True {
                n192 = invoke class="VI" method="FP.Open"(reference=w475, error in=w476, "State"=w474) -> (error out=w477:errorcluster)  [unwired: 2 in, 4 out]
              }
              frame False {
              }
            }
          }
        }
        n193 = call <vilib>:"Add State(s) to Queue__JKI_lib_State_Machine.vi"("State(s) in (\"\")"=w413) -> ("States Out"=w412:string)  [unwired: 14 in]
      }
      frame "UI: Change Zoom Factor" {
        n194 = case shown="Default" w480 {
          selector: w480 -> [_ w487]
          tunnel: [w486 w488] -> w481
          frame "" {
            n195 = local read "Zoom Factor"() -> (w486:dbl)
          }
          frame Default {
            n196 = Fract/Exp String To Number(string=w487) -> (number=w488:dbl)  [unwired: 3 in, 1 out]
          }
        }
        n197 = control-ref of="Preview"() -> (w479:refnum<vi>)
        n198 = property class="Pict"(reference=w479, "ZoomFactor"=w481) -> ()  [unwired: 1 in, 2 out]
      }
      frame "---------- Macro ----------" {
        # "Do not put any code in this frame.\n(It is a separator no-op. You can make a copy of this frame to create a new Macro frame)"
        n199 = call <vilib>:"Add State(s) to Queue__JKI_lib_State_Machine.vi"("State(s) in (\"\")"=w493) -> ("States Out"=w492:string)  [unwired: 14 in]
      }
      frame "Macro: Initialize" {
        # "Initialization Macro\n(This is called once, when the VI starts)"
        n200 = call <vilib>:"Add State(s) to Queue__JKI_lib_State_Machine.vi"("State(s) in Front (\"\")"="Data: Initialize\nInitialize Core Data\nUI: Initialize\nUI: Populate Example Tree\nUI: Initialize Panel\nUI: Front Panel State >> Open", "State(s) in (\"\")"=w499) -> ("States Out"=w498:string)  [unwired: 13 in]
      }
      frame "Macro: Exit" {
        # "Exit Macro\n(This is called once, when the VI exits)"
        n201 = Unbundle By Name(w507) -> ("Core.Close Panel on Exit?"=w506:bool)
        n202 = Select(t="UI: Front Panel State >> Close", s=w506, f="") -> (s? t:f=w503:string)
        n203 = call <vilib>:"Add State(s) to Queue__JKI_lib_State_Machine.vi"("State(s) in (\"\")"=w503, "State(s) at Back (\"\")"="Data: Cleanup\nExit") -> ("States Out"=w501:string)  [unwired: 13 in]
        n204 = call <vilib>:"Add State(s) to Queue__JKI_lib_State_Machine.vi"("State(s) in Front (\"\")"=w501, "State(s) in (\"\")"=w510) -> ("States Out"=w509:string)  [unwired: 13 in]
      }
      frame "---------- New Category ----------" {
        # "Template Separator\n(You can make a copy of, or modify, this frame)"
        n205 = call <vilib>:"Add State(s) to Queue__JKI_lib_State_Machine.vi"("State(s) in (\"\")"=w515) -> ("States Out"=w514:string)  [unwired: 14 in]
      }
      frame "New Category: 1" {
        n206 = call <vilib>:"Add State(s) to Queue__JKI_lib_State_Machine.vi"("State(s) in (\"\")"=w520) -> ("States Out"=w519:string)  [unwired: 14 in]
      }
      frame "Action: Get Bookmarks" {
        n207 = Unbundle By Name(w529) -> ("root"=w528:path)
        n208 = Build Path(base path=w528, name or relative path=w527) -> (appended path=w526:path)
        n209 = invoke class="App" method="Get VI.Bookmarks"("VIPath"=w526) -> ("BookmarkInfo"=w525:T14)  [unwired: 4 in, 4 out]
        n210 = Reverse 1D Array(array=w525) -> (reversed array=w524:T14)
        n211 = for {
          tunnel: w524 -> [w543] mode=indexing
          tunnel: [w540] -> w523 mode=indexing
          n212 = Unbundle(w543) -> ("Bookmark Reference"=w542:u32, "Bookmark Tag"=w539:string, "Label Text"=w538:string)
          n213 = call-poly <userlib>:"Convert EOLs__ogtk.vi"("Convert to:"=enum16{"CR", "LF", "CRLF"}."CR", "String in"=w538) -> ("String out"=w534:string)  [unwired: 9 in]
          n214 = call "String to 1D Array_csm.vi"("delimiter (Tab)"="\r", "string"=w534) -> ("Array of Strings"=w536:string[])  [unwired: 9 in]
          n215 = Format Into String(w542) -> (resulting string=w541:string)  [unwired: 3 in, 1 out]
          n216 = Index Array(array=w536) -> (element=w535:string)  [unwired: 1 in]
          n217 = Build Array(w535, w541, w539) -> (w540:string[])
        }
        n218 = call "Sort 2D Array.vim"("index"=0, "2D array"=w523) -> ("sorted 2D array"=w522:string[][])  [unwired: 8 in, 1 out]
        n219 = property on="BookmarkList" class="MCListbox (strict)"("ItemNames"=w522) -> ()  [unwired: 2 in, 2 out]
      }
      frame "New Category: 2" {
        # "Your code here.\n(You can make a copy of, or modify, this frame)"
        n220 = call <vilib>:"Add State(s) to Queue__JKI_lib_State_Machine.vi"("State(s) in (\"\")"=w548) -> ("States Out"=w547:string)  [unwired: 14 in]
      }
    }
  }
  n221 = call <vilib>:"Simple Error Handler.vi"("error in (no error)"=w1) -> ("error out"=w6:errorcluster)  [unwired: 4 in, 4 out]
  n222 = disable-structure shown="Disabled" {
    disable-tunnel: w6 -> [w549 _]
    frame Disabled {
      n223 = invoke class="VI" method="FP.Close"(error in=w549) -> ()  [unwired: 2 in, 3 out]
    }
    frame Enabled {
    }
  }
